vi "Get Control Information.vi"(8 "error in (no error)":errorcluster, 11 "Listbox in":refnum<class "Slide.lvclass">) -> (0 "error out":errorcluster, 2 "Control Information":string[][](array[string]), 3 "Listbox out":refnum<class "Slide.lvclass">)   [LabVIEW 2017, in "Localization.lvlib" / "Slide.lvclass"]
doc: "VI for override that is supposed to do go throgh the process for each control type and pull out the information that is necessary for each control.\n\nChoose Movement Consulting, LLC"
uses:
  Slide.lvclass
  C:/Apps/CMC/OpenSource/Localization/Control Info/Control Info.lvclass
  Localization.lvlib
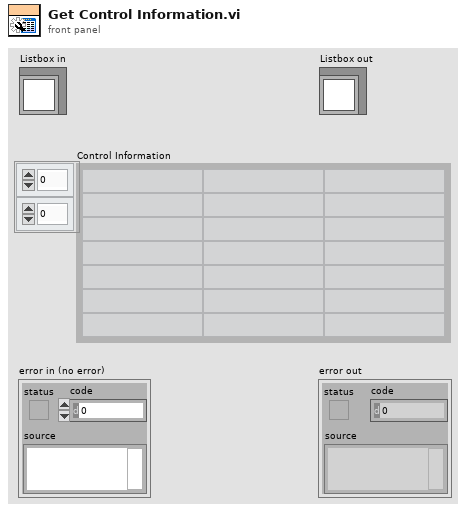
[diagram p1: front panel]
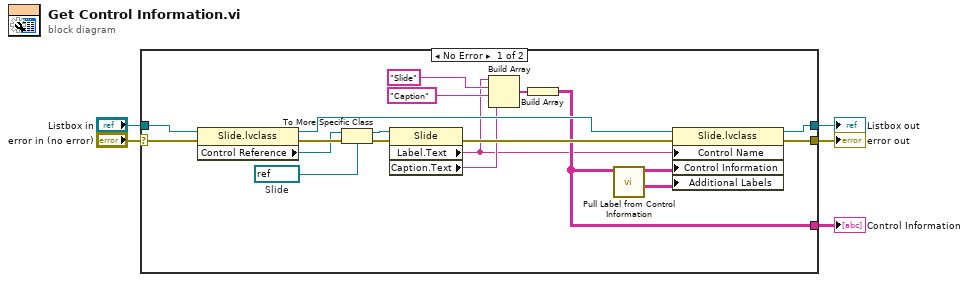
[diagram p0: block diagram]
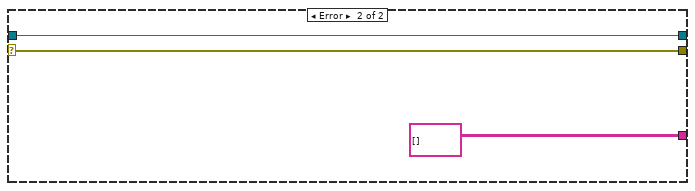
[diagram p2: hidden frame]
diagram:
  n1 = case shown="No Error" "error in (no error)" {
    selector: "error in (no error)" -> [w19 w27]
    tunnel: [w15 w27] -> w2
    tunnel: "Listbox in" -> [w18 w26]
    tunnel: [w12 string[][] []] -> w3
    tunnel: [w13 w26] -> w1
    frame No Error {
      w24 = refnum<vi> refnum  # Slide
      n2 = property class="Slide.lvclass"(reference=w18, error in=w19) -> (reference out=w14:refnum<class "Slide.lvclass">, error out=w20:errorcluster, "Control Reference"=w17:refnum<vi>)
      n3 = To More Specific Class(target class=w24, reference=w17, error in=w20) -> (specific class reference=w23:refnum<vi>, error out=w21:errorcluster)
      n4 = property class="Slide"(reference=w23, error in=w21) -> (error out=w16:errorcluster, "Label.Text"=w6:string, "Caption.Text"=w9:string)  [unwired: 1 out]
      n5 = Build Array(w6, "Slide", "Caption", w9) -> (w22:string[])
      n6 = Build Array(w22) -> (w12:string[][])
      n7 = call "Pull Label from Control Information.vi"("Control Caption Table"=w12) -> ("Additional Labels"=w7:string[][], "Control Information"=w8:string[][])  [unwired: 9 in]
      n8 = property class="Slide.lvclass"(reference=w14, error in=w16, "Control Name"=w6, "Control Information"=w8, "Additional Labels"=w7) -> (reference out=w13:refnum<class "Slide.lvclass">, error out=w15:errorcluster)
    }
    frame Error {
    }
  }
  "error out" <- w2
  "Listbox out" <- w1
  "Control Information" <- w3
